vi "Find IOV Index by Object Index.vi"(6 "Object Index":i32[](array[numeric]) format="%.0x", 7 "Address (localhost)":string="localhost", 8 "error in (no error)":errorcluster, 9 "ECAT Variables In":refnum<k21>[](array[refnum]), 10 "Slave Position Address":i32, 11 "Master ID":i32) -> (0 "error out":errorcluster, 2 "Found":bool, 3 "IOV Indeces":i32[](array[numeric]))   [LabVIEW 2016]
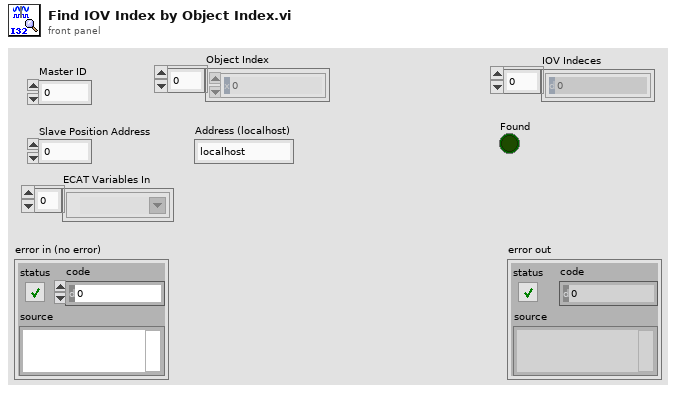
[diagram p1: front panel]
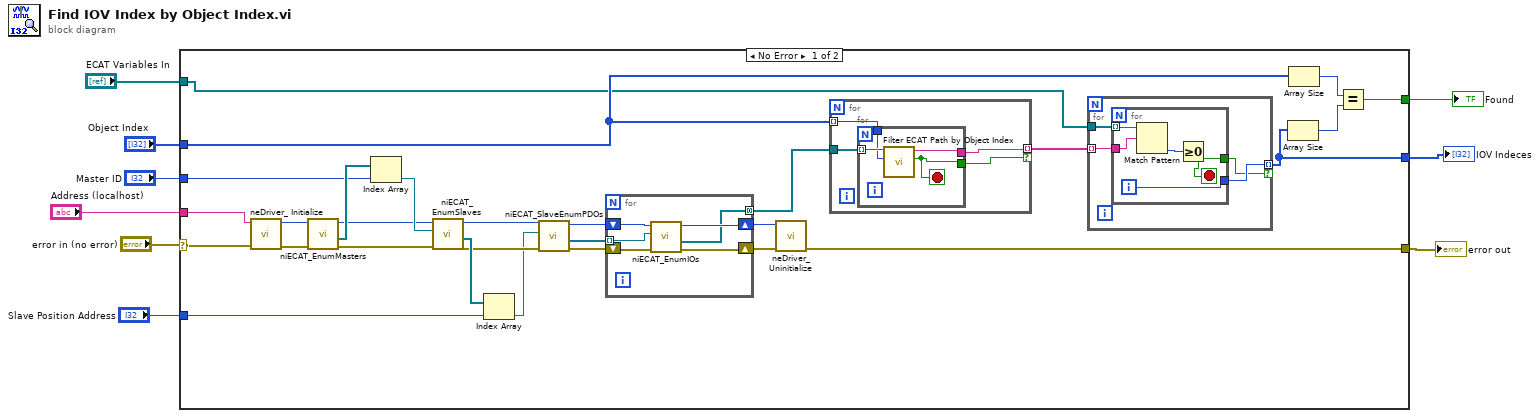
[diagram p0: block diagram]
diagram:
  n1 = case shown="No Error" "error in (no error)" {
    selector: "error in (no error)" -> [w37 _]
    tunnel: "Master ID" -> [w33 _]
    tunnel: "Slave Position Address" -> [w29 _]
    tunnel: "Object Index" -> [w18 _]
    tunnel: [w17 _] -> w5
    tunnel: "ECAT Variables In" -> [w15 _]
    tunnel: [w12 _] -> w3
    tunnel: [w11 _] -> w2
    tunnel: "Address (localhost)" -> [w10 _]
    frame No Error {
      n2 = call <vilib>:"neDriver_ Initialize.vi"("error in (no error)"=w37, "serverName"=w10) -> ("error out"=w35:errorcluster, "hServer Out"=w36:u64)  [unwired: 8 in]
      n3 = call <vilib>:"niECAT_EnumMasters.vi"("error in (no error)"=w35, "hServer In"=w36) -> ("error out"=w28:errorcluster, "masterRefs"=w34:refnum<k21>[], "hServer Out"=w31:u64)  [unwired: 7 in]
      n4 = Index Array(array=w34, index=w33) -> (element=w32:refnum<k21>)
      n5 = call <vilib>:"niECAT_EnumSlaves.vi"("error in (no error)"=w28, "Master Ref In"=w32, "hServer In"=w31) -> ("error out"=w26:errorcluster, "slaveRefs"=w30:refnum<k21>[], "hServer Out"=w27:u64)  [unwired: 5 in, 1 out]
      n6 = Index Array(array=w30, index=w29) -> (element=w25:refnum<k21>)
      n7 = call <vilib>:"niECAT_SlaveEnumPDOs.vi"("error in (no error)"=w26, "Slave Ref In"=w25, "hServer In"=w27) -> ("error out"=w23:errorcluster, "pdoRefs"=w24:refnum<k21>[], "hServer Out"=w22:u64)  [unwired: 5 in, 1 out]
      n8 = for {
        tunnel: w24 -> [w58] mode=indexing
        shift-right: [w56] -> w20
        shift-left: w23 -> [w60]
        shift-right: [w57] -> w21
        shift-left: w22 -> [w59]
        tunnel: [w55] -> w19 mode=concatenating
        n9 = call <vilib>:"niECAT_EnumIOs.vi"("error in (no error)"=w60, "PDO Ref In"=w58, "hServer In"=w59) -> ("error out"=w56:errorcluster, "IORefs"=w55:refnum<k21>[], "hServer Out"=w57:u64)  [unwired: 5 in, 1 out]
      }
      n10 = call <vilib>:"neDriver_Uninitialize.vi"("error in (no error)"=w20, "hServer In"=w21) -> ("error out"=w17:errorcluster)  [unwired: 9 in]
      n11 = for {
        tunnel: w19 -> [w50]
        tunnel: w18 -> [w49] mode=indexing
        tunnel: [w48] -> w16 mode=indexing if=w47
        n12 = for {
          tunnel: w50 -> [w54] mode=indexing
          tunnel: w49 -> [w53]
          tunnel: [w52] -> w48
          tunnel: [w51] -> w47
          stop <- w51 stop-if-true
          n13 = call "Filter ECAT Path by Object Index.vi"("Object Index In"=w53, "ECAT Variable Path In"=w54) -> ("Found"=w51:bool, "Variable Name"=w52:string)  [unwired: 8 in]
        }
      }
      n14 = for {
        tunnel: w16 -> [w40] mode=indexing
        tunnel: w15 -> [w41]
        tunnel: [w39] -> w11 mode=indexing if=w38
        n15 = for {
          tunnel: w41 -> [w45] mode=indexing
          tunnel: w40 -> [w46]
          tunnel: [w43] -> w39
          tunnel: [w42] -> w38
          i -> [w43]
          stop <- w42 stop-if-true
          n16 = Match Pattern(string=w45, regular expression=w46) -> (offset past match=w44:i32)  [unwired: 1 in, 3 out]
          n17 = Greater Or Equal To 0?(x=w44) -> (x >= 0?=w42:bool)
        }
      }
      n18 = Array Size(array=w11) -> (size(s)=w13:i32)
      n19 = Array Size(array=w18) -> (size(s)=w14:i32)
      n20 = Equal?(x=w14, y=w13) -> (x = y?=w12:bool)
    }
    frame Error {
    }
  }
  "error out" <- w5
  "IOV Indeces" <- w2
  "Found" <- w3
